vi "Data Processing Module.vi"(8 "error in (no error)":errorcluster, 9 "File Handling":refnum<queue>, 10 "UI":refnum<queue>, 11 "Queue in":refnum<queue>) -> (0 "error out":errorcluster)   [LabVIEW 2020]
uses:
  Libraries/Message Queue/Message Cluster.ctl
  <vilib>/Utility/error.llb/Error Cluster From Error Code.vi
  <vilib>/ErrorRing/Error Ring.xnode
  Libraries/Message Queue/Enqueue Message (Single).vi
  Libraries/Message Queue/Message Queue.lvlib
  Controls/Data Process Data.ctl
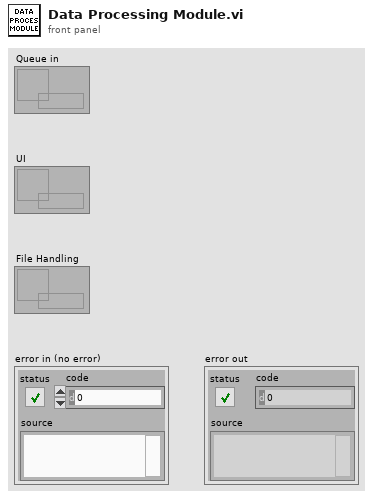
[diagram p1: front panel]
types:
  T1 = typedef "Data Process Data.ctl" = cluster{"Boolean <Replace Me>":bool, "String <Replace Me>":string, "Numeric <Replace Me>":dbl, "Do Something Ref":refnum<vi>, "Do Something Else Ref":refnum<vi>, "Data Display Ref":refnum<vi>, "Exit Button Ref":refnum<vi>}
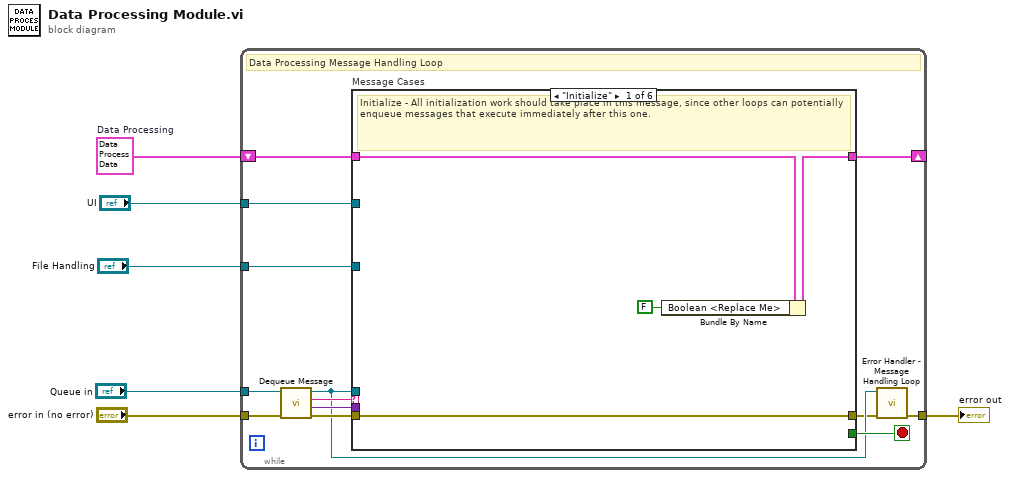
[diagram p0: block diagram]
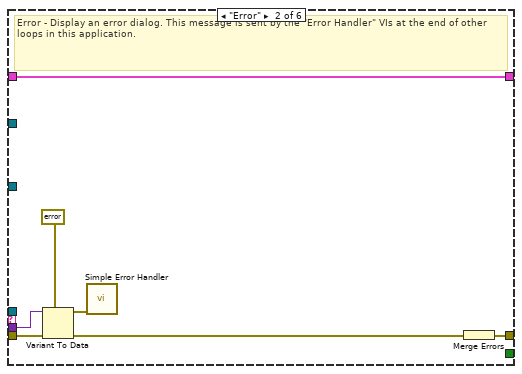
[diagram p2: hidden frame]
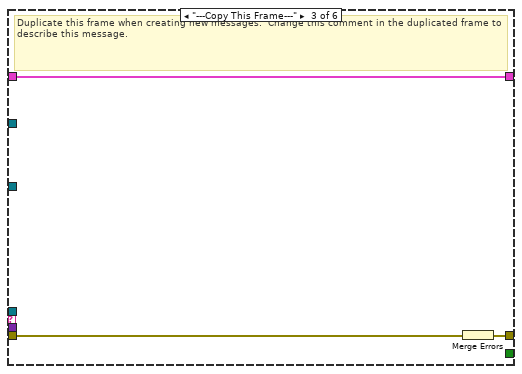
[diagram p3: hidden frame]
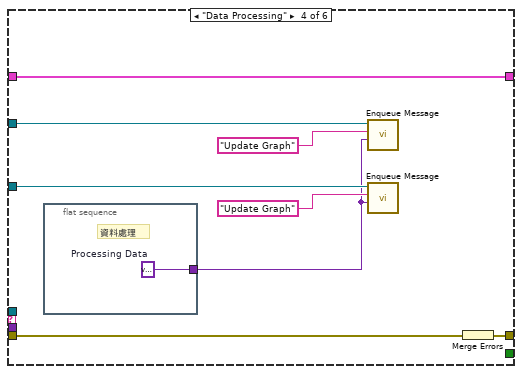
[diagram p4: hidden frame]
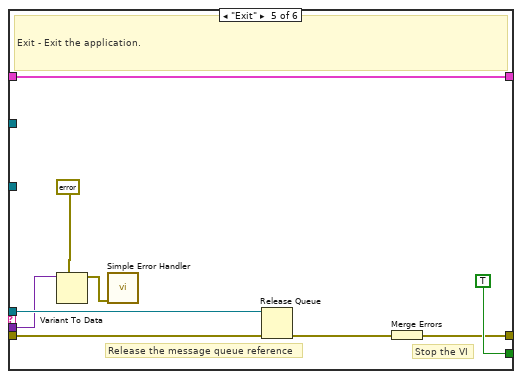
[diagram p5: hidden frame]
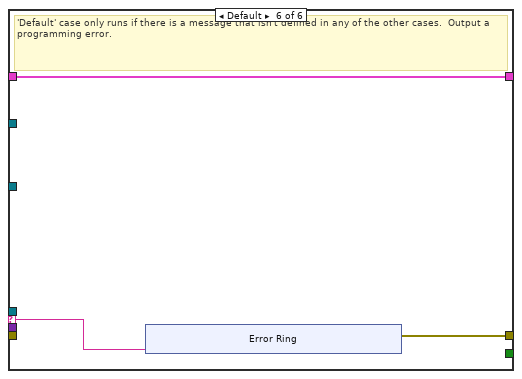
[diagram p6: hidden frame]
diagram:
  w1 = T1 {"Boolean <Replace Me>"=FALSE, "String <Replace Me>"="", "Numeric <Replace Me>"=0.0, "Do Something Ref"=refnum, "Do Something Else Ref"=refnum, "Data Display Ref"=refnum, "Exit Button Ref"=refnum}  # Data Processing
  n1 = while {
    tunnel: "Queue in" -> [w12]
    shift-right: [w18] -> _
    shift-left: w1 -> [w19]
    tunnel: "error in (no error)" -> [w16]
    tunnel: [w10] -> w5
    tunnel: "UI" -> [w8]
    tunnel: "File Handling" -> [w7]
    stop <- w17 stop-if-true
    # "Data Processing Message Handling Loop"
    n2 = call "Dequeue Message.vi"("error in (no error)"=w16, "Message Queue"=w12) -> ("error out"=w15:errorcluster, "Message Data"=w13:variant, "Message"=w14:string, "dup Message Queue"=w11:refnum<queue>)  [unwired: 6 in]
    n3 = case "Message Cases" shown="\"Initialize\"" w14 {
      selector: w14 -> [_ _ _ _ _ w52]
      tunnel: w11 -> [_ _ _ _ w51 _]
      tunnel: w15 -> [w23 w30 w33 w41 w47 _]
      tunnel: [w23 w24 w31 w39 w48 w53] -> w9
      tunnel: w19 -> [w22 w29 w32 w40 w43 w54]
      tunnel: [w21 w29 w32 w40 w43 w54] -> w18
      tunnel: [_ _ _ _ TRUE _] -> w17
      tunnel: w13 -> [_ w28 _ _ w44 _]
      tunnel: w8 -> [_ _ _ w38 _ _]
      tunnel: w7 -> [_ _ _ w35 _ _]
      frame "Initialize" {
        # "Initialize - All initialization work should take place in this message, since other loops can potentially enqueue messages that execute immediately after this one."
        n4 = Bundle By Name(cluster=w22, "Boolean <Replace Me>"=FALSE) -> (w21:T1)
      }
      frame "Error" {
        # "Error - Display an error dialog. This message is sent by the \"Error Handler\" VIs at the end of other loops in this application."
        n5 = Variant To Data(error in=w30, type=errorcluster {"status"=FALSE, "code"=0, "source"=""} ("error constant"), Variant=w28) -> (data=w26:errorcluster, error out=w25:errorcluster)
        n6 = call <vilib>:"Simple Error Handler.vi"("error in (no error)"=w26) -> ()  [unwired: 4 in, 5 out]
        n7 = Merge Errors(w25) -> (w24:errorcluster)
      }
      frame "---Copy This Frame---" {
        # "Duplicate this frame when creating new messages.  Change this comment in the duplicated frame to describe this message."
        n8 = Merge Errors(w33) -> (w31:errorcluster)
      }
      frame "Data Processing" {
        n9 = flat-sequence {
          tunnel: [w42] -> w34
          frame #0 {
            w42 = variant  # Processing Data
            # "資料處理"
          }
        }
        n10 = call-poly "Enqueue Message.vi"("Message Data"=w34, "Message"="Update Graph", "Message Queue"=w38) -> ()  [unwired: 7 in, 2 out]
        n11 = call-poly "Enqueue Message.vi"("Message Data"=w34, "Message"="Update Graph", "Message Queue"=w35) -> ()  [unwired: 7 in, 2 out]
        n12 = Merge Errors(w41) -> (w39:errorcluster)
      }
      frame "Exit" {
        # "Stop the VI"
        # "Release the message queue reference"
        # "Exit - Exit the application."
        n13 = Variant To Data(type=errorcluster {"status"=FALSE, "code"=0, "source"=""} ("error constant"), Variant=w44) -> (data=w45:errorcluster)  [unwired: 1 in, 1 out]
        n14 = call <vilib>:"Simple Error Handler.vi"("error in (no error)"=w45) -> ()  [unwired: 4 in, 5 out]
        n15 = Release Queue(queue=w51, error in (no error)=w47) -> (error out=w49:errorcluster)  [unwired: 1 in, 2 out]
        n16 = Merge Errors(w49) -> (w48:errorcluster)
      }
      frame Default {
        # "'Default' case only runs if there is a message that isn't defined in any of the other cases.  Output a programming error."
        n17 = xnode "Error Ring"("parameter 0"=w52) -> ("error out"=w53:errorcluster)
      }
    }
    n18 = call "Error Handler - Message Handling Loop.vi"("error in (no error)"=w9, "Message Queue"=w11) -> ("dup error in"=w10:errorcluster)  [unwired: 8 in, 1 out]
  }
  "error out" <- w5
